vi "PCAN_DecompMessage.vi"(11 "CAN_Message out":T1) -> (0 "Intensity (a.u.)":dbl, 1 "Detector2 Shutter Open?":bool, 2 "Detector1 Shutter Open?":bool, 3 "Excitation Shutter Open?":bool, 4 "Laser 1-4":u8[](array[numeric]), 6 "Laser 5-8":u8[](array[numeric]))   [LabVIEW 2009]
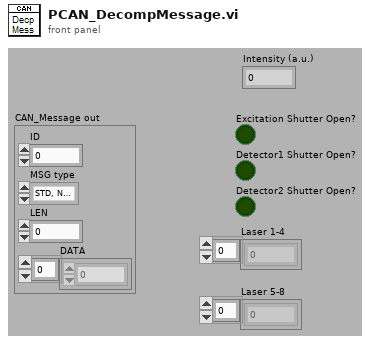
[diagram p1: front panel]
types:
  T1 = cluster{"ID":u32, "MSG type":enum8{"STD, NO RTR", "STD,RTR", "XTD, NO RTR", "XTD, RTR"}, "LEN":u8, "DATA":u8[]}
  T2 = enum8{"STD, NO RTR", "STD,RTR", "XTD, NO RTR", "XTD, RTR"}
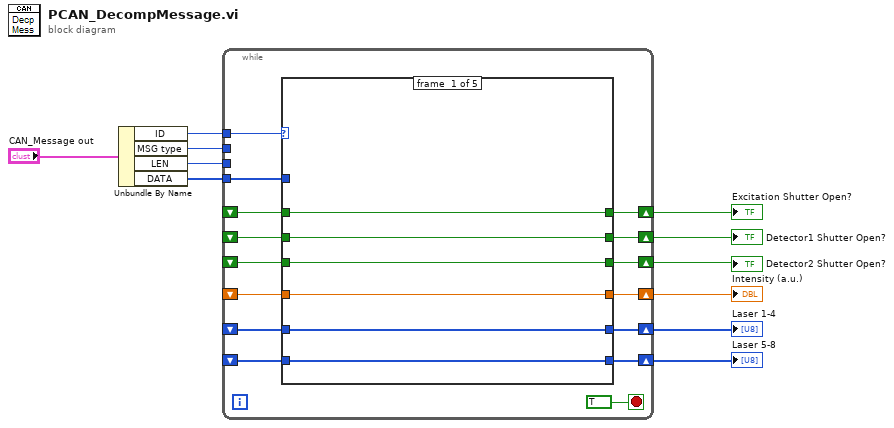
[diagram p0: block diagram]
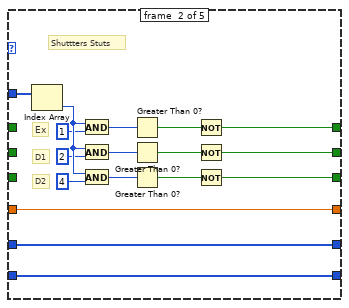
[diagram p2: hidden frame]
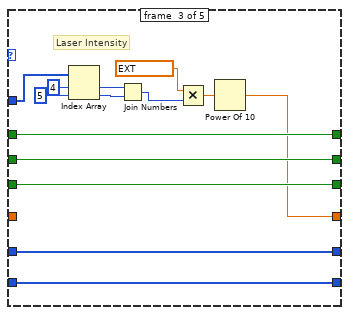
[diagram p3: hidden frame]
diagram:
  n1 = Unbundle By Name("CAN_Message out") -> ("ID"=w10:u32, "MSG type"=w9:T2, "LEN"=w8:u8, "DATA"=w7:u8[])
  n2 = while {
    tunnel: w10 -> [w25]
    tunnel: w9 -> [_]
    tunnel: w8 -> [_]
    tunnel: w7 -> [w24]
    shift-right: [w23] -> w5
    shift-left: _ -> [w18]
    shift-right: [w22] -> w4
    shift-left: _ -> [w19]
    shift-right: [w21] -> w6
    shift-left: _ -> [w20]
    shift-right: [w17] -> w3
    shift-left: _ -> [w16]
    shift-right: [w15] -> w2
    shift-left: _ -> [w14]
    shift-right: [w13] -> w1
    shift-left: _ -> [w12]
    stop <- TRUE stop-if-true
    n3 = case shown="1793" w25 {
      tunnel: w24 -> [_ w49 w60 w65 w70]
      tunnel: [w30 w38 w61 w67 w73] -> w23
      tunnel: [w31 w37 w62 w68 w74] -> w22
      tunnel: [w32 w36 w63 w69 w75] -> w21
      tunnel: w20 -> [w32 _ w63 w69 w75]
      tunnel: w19 -> [w31 _ w62 w68 w74]
      tunnel: w18 -> [w30 _ w61 w67 w73]
      tunnel: [w29 w35 w53 w66 w72] -> w17
      tunnel: w16 -> [w29 w35 _ w66 w72]
      tunnel: [w28 w34 w51 w65 w71] -> w15
      tunnel: w14 -> [w28 w34 w51 _ w71]
      tunnel: [w27 w33 w50 w64 w70] -> w13
      tunnel: w12 -> [w27 w33 w50 w64 _]
      frame #0 {
      }
      frame #1 {
        # "Shuttters Stuts"
        # "D2"
        # "D1"
        # "Ex"
        n4 = Index Array(array=w49) -> (element=w48:u8)  [unwired: 1 in]
        n5 = And(x=w48, y=u8 1) -> (x .and. y?=w44:u8)
        n6 = And(x=w48, y=u8 2) -> (x .and. y?=w43:u8)
        n7 = And(x=w48, y=u8 4) -> (x .and. y?=w42:u8)
        n8 = Greater Than 0?(x=w44) -> (x > 0?=w41:bool)
        n9 = Greater Than 0?(x=w43) -> (x > 0?=w40:bool)
        n10 = Greater Than 0?(x=w42) -> (x > 0?=w39:bool)
        n11 = Not(x=w41) -> (.not. x?=w36:bool)
        n12 = Not(x=w40) -> (.not. x?=w37:bool)
        n13 = Not(x=w39) -> (.not. x?=w38:bool)
      }
      frame #2 {
        # "Laser Intensity"
        n14 = Index Array(array=w60, index #1=4 ("index"), index #2=5 ("index")) -> (element #1=w57:u8, element #2=w56:u8)
        n15 = Join Numbers(hi=w57, lo=w56) -> ((hi.lo)=w52:u16)
        n16 = Multiply(x=ext 0.0097752, y=w52) -> (x*y=w54:ext)
        n17 = Power Of 10(x=w54) -> (10^x=w53:ext)
      }
      frame #3 {
        # "Laser Controler 1"
      }
      frame #4 {
        # "Laser Controler 2"
      }
    }
  }
  "Excitation Shutter Open?" <- w6
  "Detector2 Shutter Open?" <- w5
  "Detector1 Shutter Open?" <- w4
  "Intensity (a.u.)" <- w3
  "Laser 1-4" <- w2
  "Laser 5-8" <- w1
